vi "Configure Baseband Frequency Offset.vi"(8 "error in (no error)":errorcluster, 9 "Baseband Frequency Offset (0 Hz)":dbl, 10 "Modulation Format (1: Dual Modulation)":u16(ring)=1 items=["Custom"=0, "Dual Modulation"=1, "Dual ARB"=2, "Multitone"=3, "Two-tone"=6], 11 "VISA resource name":refnum<visa-resource-name>) -> (0 "error out":errorcluster, 3 "VISA resource name out":refnum<visa-resource-name>)   [LabVIEW 2018, in "Agilent PSG MXG Series.lvlib"]
doc: "Configures baseband frequency offset.\n\n<B>Notes:</B>\n(1) This VI is valid only in N5172B, N5182B, N5162A/82A that install <B>Option 651</B> or <B>Option 652</B> or <B>Option 654</B> (Internal baseband generator)."
uses:
  Agilent PSG MXG Series.lvlib
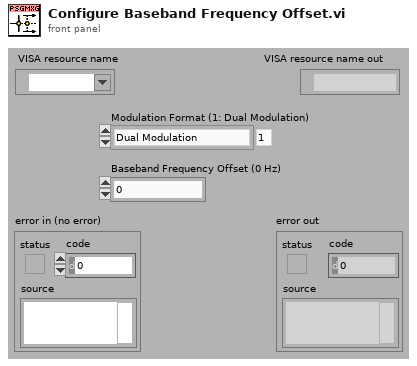
[diagram p1: front panel]
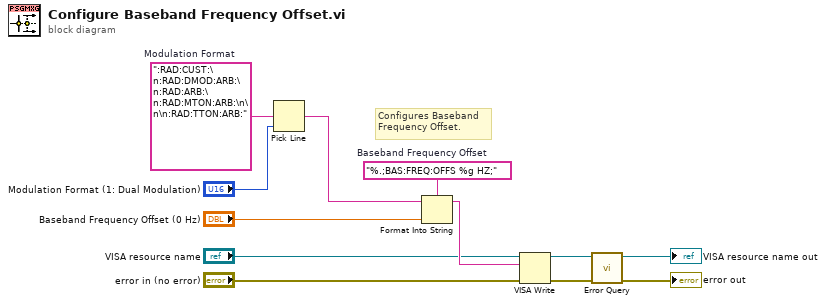
[diagram p0: block diagram]
diagram:
  w10 = "%.;BAS:FREQ:OFFS %g HZ;"  # Baseband Frequency Offset
  w12 = ":RAD:CUST:\n:RAD:DMOD:ARB:\n:RAD:ARB:\n:RAD:MTON:ARB:\n\n\n:RAD:TTON:ARB:"  # Modulation Format
  # "Configures Baseband\nFrequency Offset."
  n1 = Pick Line(multi-line string=w12, line index="Modulation Format (1: Dual Modulation)") -> (output string=w9:string)  [unwired: 1 out]
  n2 = Format Into String(format string=w10, initial string=w9, "Baseband Frequency Offset (0 Hz)") -> (resulting string=w7:string)  [unwired: 1 in, 1 out]
  n3 = VISA Write(VISA resource name="VISA resource name", write buffer=w7, error in (no error)="error in (no error)") -> (VISA resource name out=w6:refnum<visa-resource-name>, error out=w5:errorcluster)  [unwired: 1 out]
  n4 = call "Error Query.vi"("error in (no error)"=w5, "VISA resource name"=w6) -> ("error out"=→"error out":errorcluster, "VISA resource name out"=→"VISA resource name out":refnum<visa-resource-name>)  [unwired: 8 out]
